vi "inline_table_delete_item.vi"(7 "subtables":string[](array[string]), 8 "error in (no error)":errorcluster, 10 "key":string, 11 "InlineTable in":refnum<class "InlineTable.lvclass">) -> (0 "error out":errorcluster, 2 "removed?":bool, 3 "InlineTable out":refnum<class "InlineTable.lvclass">)   [LabVIEW 2020, in "toml.lvclass"]
uses:
  toml.lvclass
  InlineTable/InlineTable.lvclass
  toml.lvclass/toml.ctl
  Item/Item.lvclass
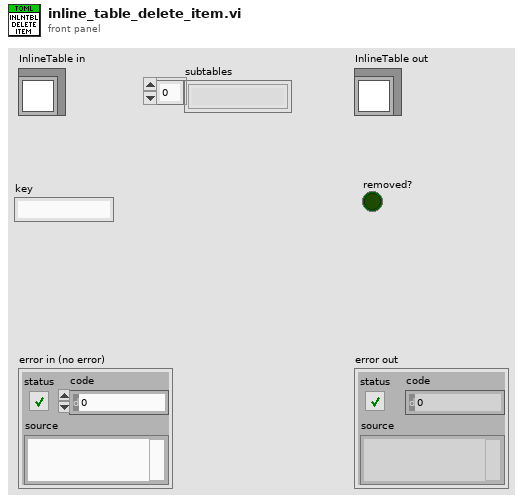
[diagram p1: front panel]
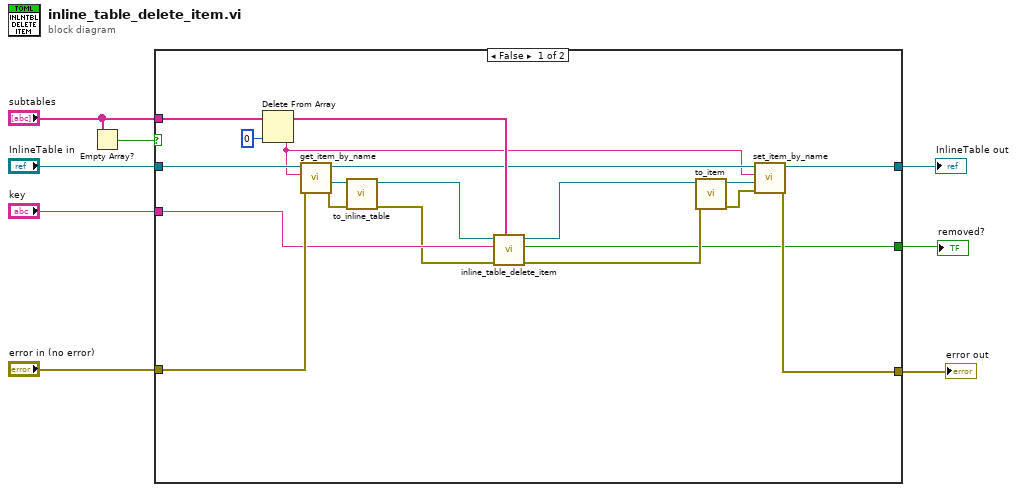
[diagram p0: block diagram]
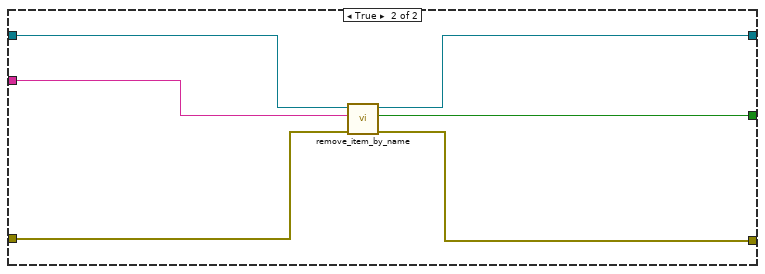
[diagram p2: hidden frame]
diagram:
  n1 = Empty Array?(array="subtables") -> (empty?=w4:bool)
  n2 = case shown="False" w4 {
    tunnel: [w21 w33] -> w8
    tunnel: [w17 w32] -> w7
    tunnel: "InlineTable in" -> [w24 w31]
    tunnel: "error in (no error)" -> [w23 w30]
    tunnel: "subtables" -> [w27 _]
    tunnel: "key" -> [w16 w29]
    tunnel: [w11 w28] -> w1
    frame False {
      n3 = Delete From Array(array=w27, index=0) -> (deleted portion=w20:string, array with subset deleted=w25:string[])  [unwired: 1 in]
      n4 = call "get_item_by_name.vi"("error in (no error)"=w23, "key_name"=w20, "Table in"=w24) -> ("error out"=w15:errorcluster, "Item"=w14:refnum<class "Item.lvclass">, "Table out"=w22:refnum<class "InlineTable.lvclass">)  [unwired: 6 in]
      n5 = call "to_inline_table.vi"("error in (no error)"=w15, "Item in"=w14) -> ("error out"=w12:errorcluster, "InlineTable"=w13:refnum<class "InlineTable.lvclass">)  [unwired: 8 in]
      n6 = call "inline_table_delete_item.vi"("subtables"=w25, "error in (no error)"=w12, "key"=w16, "InlineTable in"=w13) -> ("error out"=w18:errorcluster, "removed?"=w11:bool, "InlineTable out"=w19:refnum<class "InlineTable.lvclass">)  [unwired: 5 in]
      n7 = call "to_item.vi"("error in (no error)"=w18, "Table in"=w19) -> ("error out"=w10:errorcluster, "Item out"=w9:refnum<class "Item.lvclass">)  [unwired: 8 in]
      n8 = call "set_item_by_name.vi"("error in"=w10, "Item"=w9, "key_name"=w20, "Table in"=w22) -> ("error out"=w21:errorcluster, "Table out"=w17:refnum<class "InlineTable.lvclass">)  [unwired: 6 in]
    }
    frame True {
      n9 = call "remove_item_by_name.vi"("error in (no error)"=w30, "item_name"=w29, "InlineTable in"=w31) -> ("error out"=w33:errorcluster, "removed?"=w28:bool, "InlineTable out"=w32:refnum<class "InlineTable.lvclass">)  [unwired: 6 in]
    }
  }
  "error out" <- w8
  "InlineTable out" <- w7
  "removed?" <- w1
